vi "WriteLoopMarco.vi"() -> ()   [LabVIEW 2023]
panel:
  out "resulting string":string
  in  "Hysteresis":dbl min=-5.0 max=5.0 step=0.1
  in  "Target":dbl min=-230.0 max=50.0
  in  "Input":u16(ring) items=["3A", "3B", "3C", "3D", "4A", "4B"]
  in  "Relay":u16(ring) items=["A", "B", "C", "D"]
  in  "MacroName":u16(ring) items=["ColdLoop", "HotLoop"]
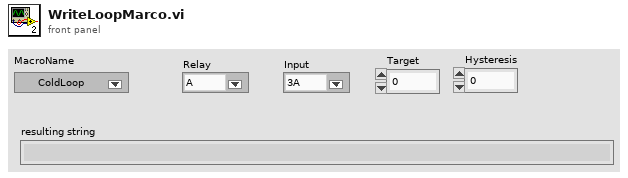
[diagram p1: front panel]
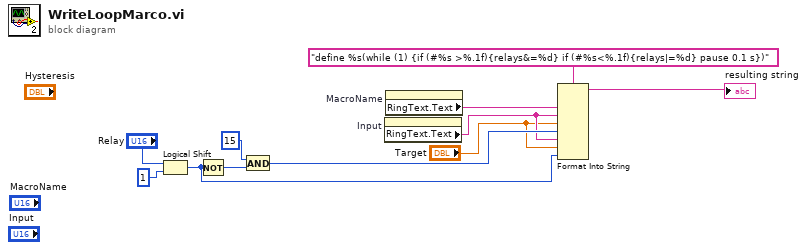
[diagram p0: block diagram]
diagram:
  n1 = Logical Shift(y="Relay", x=u8 1) -> (x << y=w1:u8)
  n2 = Not(x=w1) -> (.not. x?=w9:u8)
  n3 = And(x=u8 15, y=w9) -> (x .and. y?=w4:u8)
  n4 = property on="Input" class="Ring (strict)"() -> ("RingText.Text"=w3:string)  [unwired: 2 in, 2 out]
  n5 = property on="MacroName" class="Ring (strict)"() -> ("RingText.Text"=w6:string)  [unwired: 2 in, 2 out]
  n6 = Format Into String(format string="define %s(while (1) {if (#%s >%.1f){relays&=%d} if (#%s<%.1f){relays|=%d} pause 0.1 s})", w6, w3, "Target", w4, w3, "Target", w1) -> (resulting string=→"resulting string":string)  [unwired: 2 in, 1 out]
